vi "load wheel.vi"(8 "error in (no error)":errorcluster, 11 "file path":path) -> (0 "error out":errorcluster, 2 "cycle file path (Not A Path if cancelled)":path, 3 "Wheel run order array":string[][](array[string]), 4 "run order path":path)   [LabVIEW 2016]
doc: "This vi will load a wheel on command. It asks the user for a wheel table file and generates a run order with 2 sequences per sample and 4 samples between standards"
uses:
  <vilib>/Utility/file.llb/Read Delimited Spreadsheet (string).vi
panel:
  out "sequence path":path
  out "wheel name":string
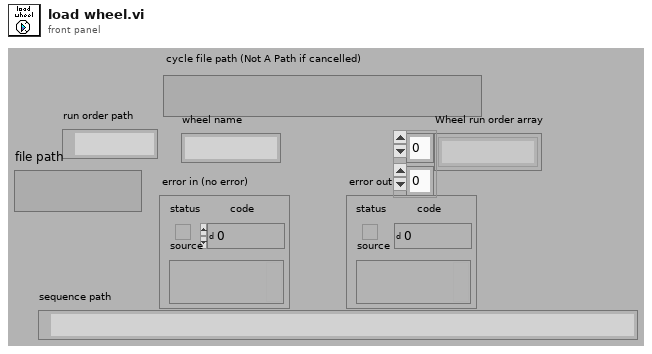
[diagram p1: front panel]
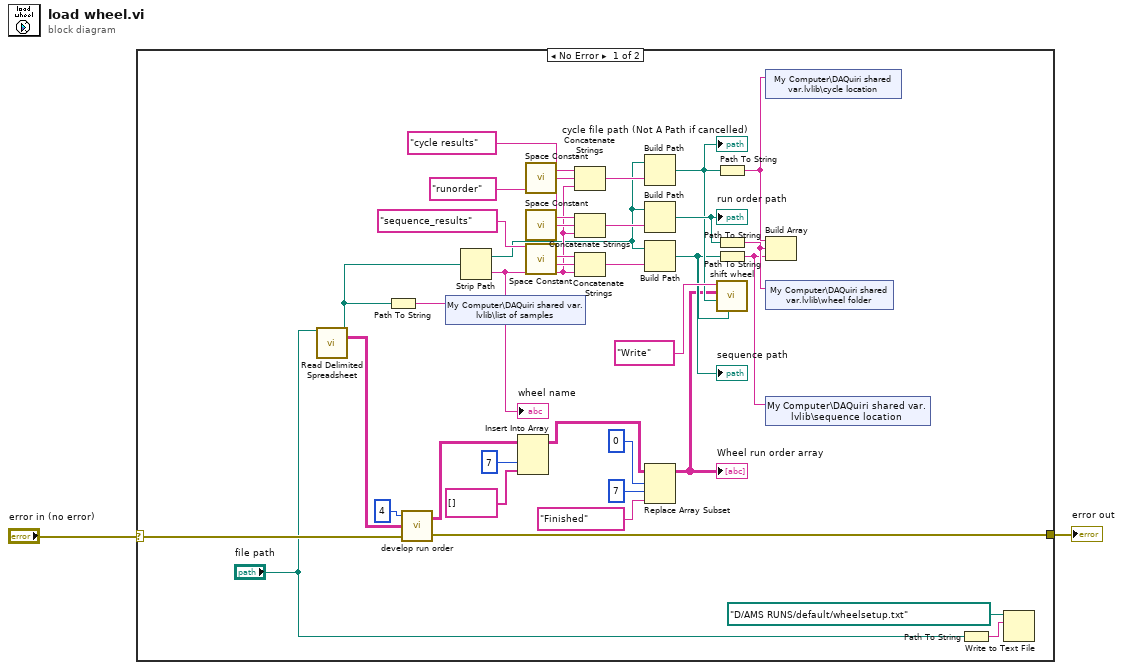
[diagram p0: block diagram]
diagram:
  n1 = case shown="No Error" "error in (no error)" {
    selector: "error in (no error)" -> [w28 w38]
    tunnel: [w29 w38] -> w2
    frame No Error {
      n2 = call-poly <vilib>:"Read Delimited Spreadsheet.vi"("file path (dialog if empty)"="file path") -> ("new file path (Not A Path if cancelled)"=w15:path, "all rows"=w3:string[][])  [unwired: 9 in, 4 out]
      n3 = Path To String(path=w15) -> (string=w16:string)
      n4 = call "develop run order.vi"("error in (no error)"=w28, "all rows"=w3, "number of samples between standards"=4) -> ("error out"=w29:errorcluster, "Group run list"=w35:string[][])
      n5 = shared-variable "My Computer\\DAQuiri shared var.lvlib\\list of samples"(w16) -> ()  [unwired: 1 in, 1 out]
      n6 = Strip Path(path=w15) -> (stripped path=w20:path, name=w21:string)
      "wheel name" <- w21
      n7 = Insert Into Array(array=w35, index (col)=7 ("disabled index (col)"), new element=string[] [] ("new element/subarray")) -> (w14:string[][])  [unwired: 1 in]
      n8 = call <vilib>:"Space Constant.vi"() -> ("String"=w31:string)
      n9 = call <vilib>:"Space Constant.vi"() -> ("String"=w23:string)
      n10 = call <vilib>:"Space Constant.vi"() -> ("String"=w27:string)
      n11 = Concatenate Strings("cycle results" ("string"), w31, w21) -> (w30:string)
      n12 = Concatenate Strings("runorder" ("string"), w23, w21) -> (w22:string)
      n13 = Concatenate Strings("sequence_results" ("string"), w27, w21) -> (w25:string)
      n14 = Build Path(base path=w20, name or relative path=w30) -> (appended path=w18:path)
      "cycle file path (Not A Path if cancelled)" <- w18
      n15 = Build Path(base path=w20, name or relative path=w22) -> (appended path=w19:path)
      "run order path" <- w19
      n16 = Build Path(base path=w20, name or relative path=w25) -> (appended path=w17:path)
      "sequence path" <- w17
      n17 = Replace Array Subset(array=w14, new element="Finished", index (row)=0, index (col)=7 ("disabled index (col)")) -> (w10:string[][])
      "Wheel run order array" <- w10
      n18 = Path To String(path=w18) -> (string=w8:string)
      n19 = Path To String(path=w19) -> (string=w7:string)
      n20 = Path To String(path=w17) -> (string=w6:string)
      n21 = call "shift wheel.vi"("seq results name in"=w17, "cycle results name in"=w18, "Group run list write"=w10, "read write"="Write") -> ()  [unwired: 5 in, 3 out]
      n22 = shared-variable "My Computer\\DAQuiri shared var.lvlib\\cycle location"(w8) -> ()  [unwired: 1 in, 1 out]
      n23 = Build Array(w8, w7, w6) -> ()  [unwired: 1 out]
      n24 = shared-variable "My Computer\\DAQuiri shared var.lvlib\\wheel folder"(w7) -> ()  [unwired: 1 in, 1 out]
      n25 = shared-variable "My Computer\\DAQuiri shared var.lvlib\\sequence location"(w6) -> ()  [unwired: 1 in, 1 out]
      n26 = Path To String(path="file path") -> (string=w4:string)
      n27 = Write to Text File(file (use dialog)=path "D:/AMS RUNS/default/wheelsetup.txt", text=w4) -> ()  [unwired: 2 in, 3 out]
    }
    frame Error {
    }
  }
  "error out" <- w2
